vi "Taller1_GeneracionDeSonido_Log.vi"() -> ()   [LabVIEW 2022 SP3]
uses:
  <vilib>/sound2/lvsound2.llb/Sampling Mode.ctl
  <vilib>/sound2/lvsound2.llb/Sound Data Format.ctl
  <vilib>/addons/_NISVFA/_Generation/Signal Generation/SV Signal/SV Signal.lvclass/SV Signal.ctl
  <vilib>/addons/_NISVFA/_Generation/Signal Generation/SV Signal/Read Total Samples.vi
  <vilib>/addons/_NISVFA/_Generation/Signal Generation/SV Signal/Calculate Number of Remaining Samples.vi
  <vilib>/addons/_NISVFA/_Generation/Signal Generation/SV Continuous Sweep/SV Continuous Sweep.lvclass
  C:/Program Files/NI/LVAddons/nisvt/1/vi.lib/addons/_NISVFA/_Generation/Signal Generation/SV Signal/SV Signal.lvclass
  <vilib>/addons/_NISVFA/_Generation/Signal Generation/SV Continuous Sweep/Configure Continuous Sweep.vi
  <vilib>/addons/_NISVFA/_Generation/Signal Generation/SV Signal/Write Sample Rate.vi
  <vilib>/addons/_NISVFA/_Generation/Signal Generation/SV Signal/Read Generation State.vi
  <vilib>/addons/_NISVFA/_Generation/Signal Generation/SV Signal/Read System Timing Model.vi
  <vilib>/addons/_NISVFA/_Generation/Signal Generation/SV Continuous Sweep/Read Frequency Waveform.vi
  <vilib>/sound2/lvsound2.llb/Sound Output Set Volume (Single).vi
  <vilib>/sound2/lvsound2.llb/Sound Output Write (DBL Single).vi
  <vilib>/addons/_NISVFA/_Generation/Signal Generation/SV Signal/SV Signal.lvclass
panel:
  in  "stop":bool
  in  "Device ID":u32
  out "Generated Sound":waveform(dbl)(graph)
  in  "Volume":dbl(slide)=50.0 scale=0.0..100.0
  out "Continuous Frequency Sweep":waveform(dbl)[](graph)
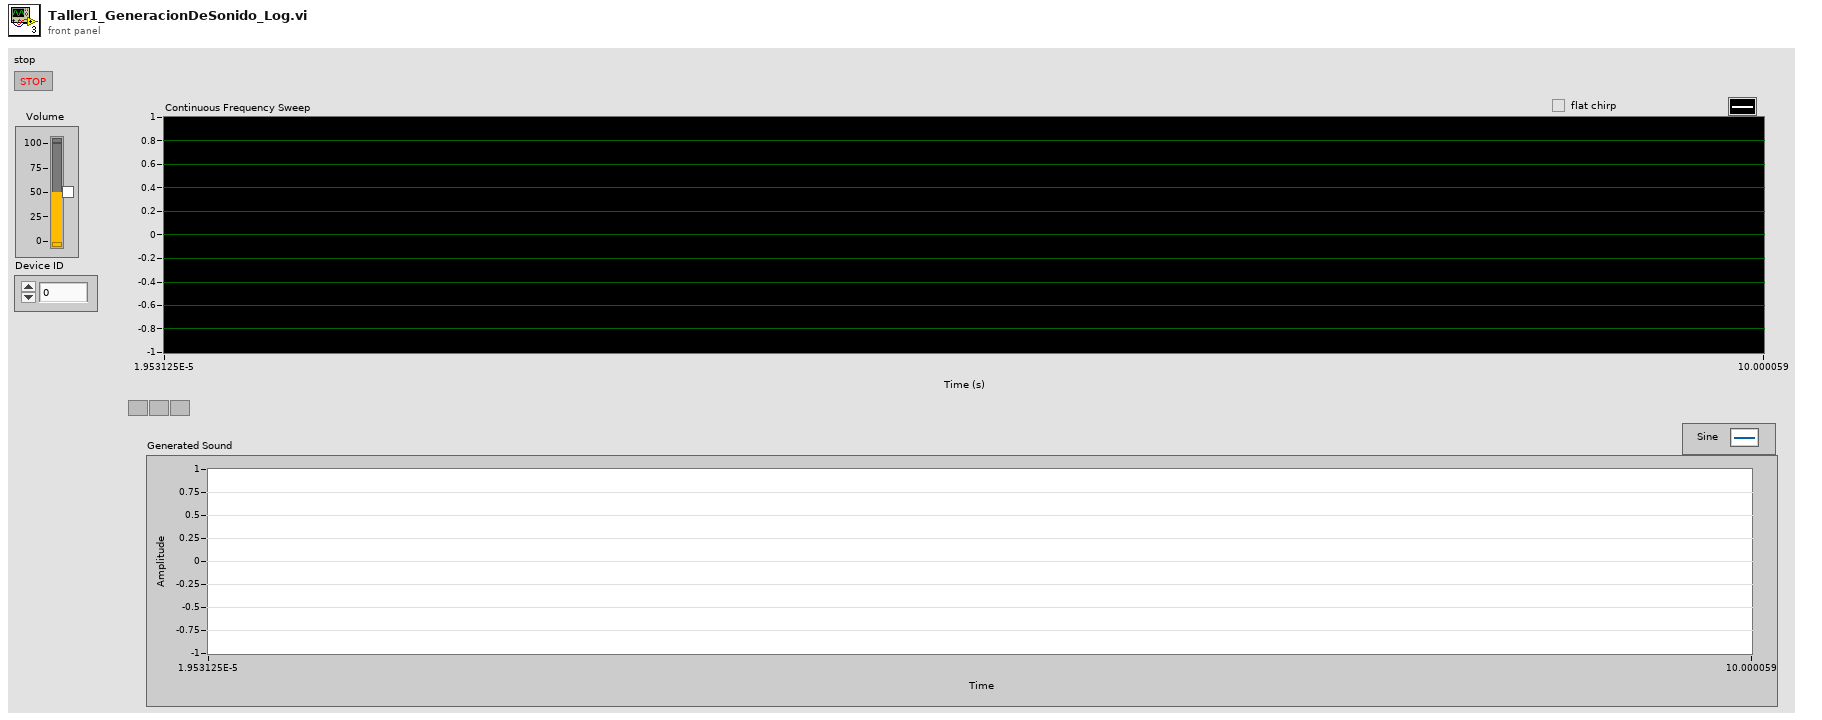
[diagram p1: front panel]
types:
  T1 = typedef "Sound Data Format.ctl" = cluster{"sample rate (S/s)":dbl, "number of channels":i32, "bits per sample":i32}
  T2 = typedef "Sampling Mode.ctl" = i32
  T3 = typedef "Sound Output Task ID.ctl" = u32
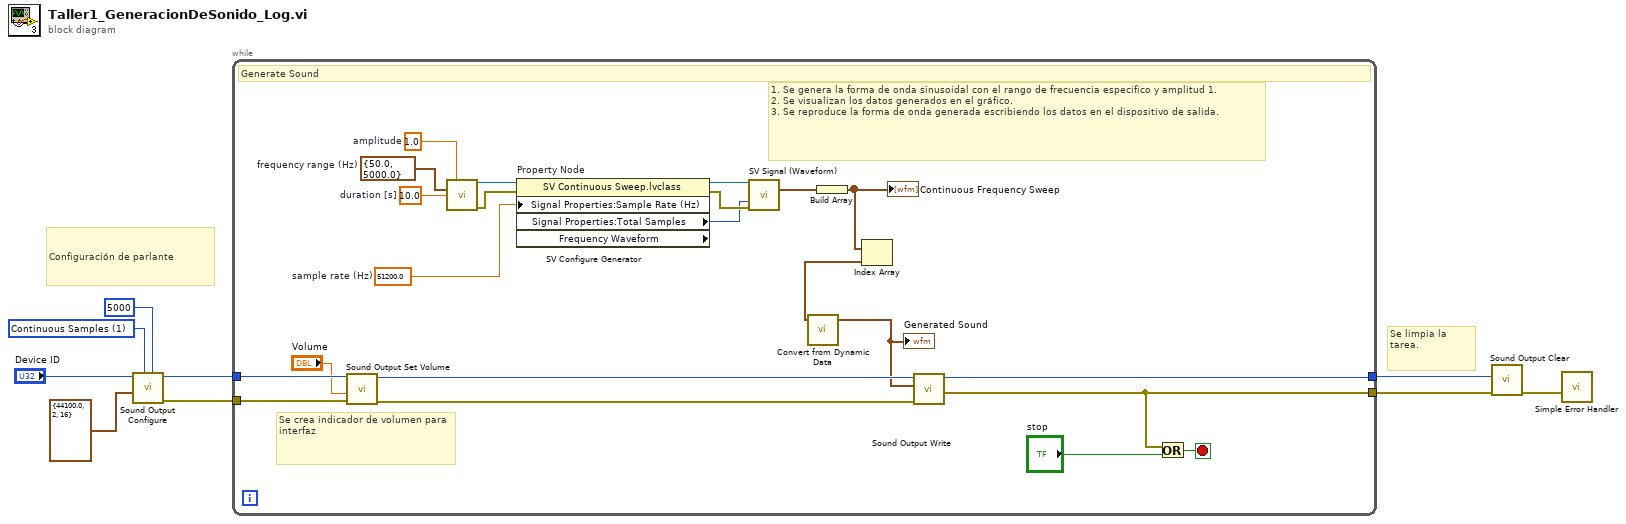
[diagram p0: block diagram]
diagram:
  w4 = T2 1 items=["Finite Samples", "Continuous Samples"] ("sample mode")
  # "Configuración de parlante"
  # "Se limpia la tarea."
  n1 = call <vilib>:"Sound Output Configure.vi"("number of samples/ch"=5000 ("Number of Samples/ch"), "sample mode"=w4, "sound format"=T1 {"sample rate (S/s)"=44100.0, "number of channels"=2, "bits per sample"=16} ("Sound Format"), "device ID"="Device ID") -> ("error out"=w9:errorcluster, "task ID"=w8:T3)  [unwired: 6 in]
  n2 = while {
    tunnel: w8 -> [w27]
    tunnel: [w31] -> w6
    tunnel: w9 -> [w29]
    tunnel: [w25] -> w7
    stop <- w30 stop-if-true
    w18 = 51200.0  # sample rate (Hz)
    w17 = 1.0  # amplitude
    w15 = 10.0  # duration [s]
    w16 = cluster{"start":dbl, "stop":dbl} {"start"=50.0, "stop"=5000.0}  # frequency range (Hz)
    # "Se crea indicador de volumen para interfaz"
    # "1. Se genera la forma de onda sinusoidal con el rango de frecuencia especifico y amplitud 1. \n2. Se visualizan los datos generados en el gráfico. \n3. Se reproduce la forma de onda generada escribiendo los datos en el dispositivo de salida."
    # "Generate Sound"
    n3 = call-poly <vilib>:"Sound Output Set Volume.vi"("error in (no error)"=w29, "volume"="Volume", "task ID"=w27) -> ("error out"=w11:errorcluster, "task ID out"=w28:T3)  [unwired: 7 in]
    n4 = call-poly <vilib>:"SV Configure Generator.vi"("amplitude"=w17, "frequency range [Hz]"=w16, "duration [s]"=w15) -> ("signal configuration"=w19:refnum<class "SV Continuous Sweep.lvclass">, "error out"=w22:errorcluster)  [unwired: 11 in]
    n5 = property on="Property Node" class="SV Continuous Sweep.lvclass" props=["Signal Properties:Sample Rate (Hz)", "Signal Properties:Total Samples", "Frequency Waveform"](reference=w19, error in=w22, "Signal Properties:Sample Rate (Hz)"=w18) -> (reference out=w20:refnum<class "SV Continuous Sweep.lvclass">, error out=w23:errorcluster, "Signal Properties:Total Samples"=w21:i32)  [unwired: 1 out]
    n6 = call-dynamic "SV Signal (Waveform).vi"("signal configuration"=w20, "samples"=w21, "error in (no error)"=w23) -> ("output waveform"=w14:waveform(dbl))  [unwired: 7 in, 5 out]
    n7 = Build Array(w14) -> (w13:waveform(dbl)[])
    "Continuous Frequency Sweep" <- w13
    n8 = Index Array(array=w13) -> (element=w12:waveform(dbl))  [unwired: 1 in]
    n9 = call "Convert from Dynamic Data"("Dynamic Data Type"=w12) -> ("Waveform"=w24:waveform(dbl))  [unwired: 3 in]
    "Generated Sound" <- w24
    n10 = call-poly <vilib>:"Sound Output Write.vi"("error in (no error)"=w11, "data"=w24, "task ID"=w28) -> ("error out"=w25:errorcluster, "task ID out"=w31:T3)  [unwired: 7 in]
    n11 = Or(x=w25, y="stop") -> (x .or. y?=w30:bool)
  }
  n12 = call <vilib>:"Sound Output Clear.vi"("error in (no error)"=w7, "task ID"=w6) -> ("error out"=w2:errorcluster)  [unwired: 9 in]
  n13 = call <vilib>:"Simple Error Handler.vi"("error in (no error)"=w2) -> ()  [unwired: 4 in, 5 out]
